vi "Read Switch Setting.vi"(8 "error in (no error)":errorcluster, 11 "Switch configuration":refnum<class "Switch configuration.lvclass">) -> (0 "error out":errorcluster, 2 "Switch Setting":T1, 3 "Switch configuration out":refnum<class "Switch configuration.lvclass">)   [LabVIEW 2025, in "Switch.lvlib" / "Switch configuration.lvclass"]
uses:
  Switch configuration.lvclass
  Switch Instrument Setting.ctl
  Switch configuration.lvclass/Switch configuration.ctl
  <instrlib>/niSwitch/niSwitch.llb/niSwitch Topologies.ctl
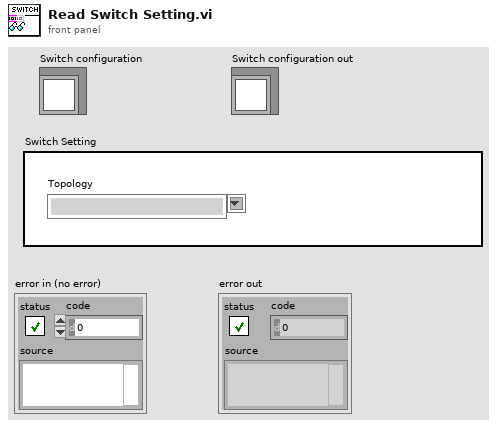
[diagram p1: front panel]
types:
  T1 = typedef "Switch.lvlib/Switch configuration.lvclass/Switch Instrument Setting.ctl" = cluster{"topology name":T2}
  T2 = typedef "niSwitch Topologies.ctl" = string
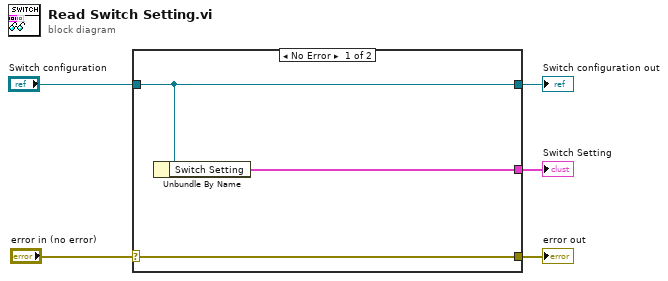
[diagram p0: block diagram]
diagram:
  n1 = case shown="No Error" "error in (no error)" {
    selector: "error in (no error)" -> [w8 w9]
    tunnel: [w8 w9] -> w4
    tunnel: [w7 w10] -> w2
    tunnel: "Switch configuration" -> [w7 w10]
    tunnel: [w6 _] -> w1
    frame No Error {
      n2 = Unbundle By Name(w7) -> ("Switch Setting"=w6:T1)
    }
    frame Error {
    }
  }
  "error out" <- w4
  "Switch configuration out" <- w2
  "Switch Setting" <- w1
